vi "GetSpeedProperties.vi"(11 "properties":T2[](array[typedef])) -> (1 "speed reference id":string, 2 "nominal speed":dbl, 3 "speed type":T1)   [LabVIEW 2017, in "VibrationAnalysis.lvlib"]
uses:
  <vilib>/addons/InsightCM/Devices/Shared/VibrationAnalysis/VibrationAnalysis.lvlib
  <vilib>/addons/InsightCM/Utilities/PropertyHelpers/PropertyHelpers.lvlib
  <vilib>/addons/InsightCM/Utilities/Analysis/Shared/controls/SpeedType.ctl
  <vilib>/addons/InsightCM/Utilities/Analysis/Shared/AnalysisHelper.lvlib
  <vilib>/addons/InsightCM/MessageBus/Base/controls/KeyValuePair.ctl
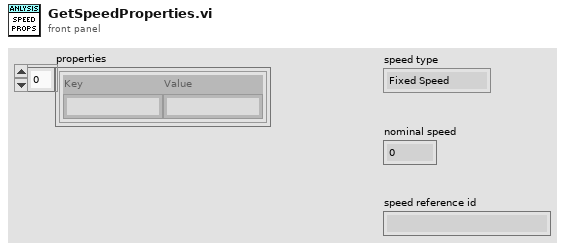
[diagram p1: front panel]
types:
  T1 = typedef "AnalysisHelper.lvlib/SpeedType.ctl" = enum16{"Fixed Speed", "Tachometer"}
  T2 = typedef "KeyValuePair.ctl" = cluster{"Key":string, "Value":string}
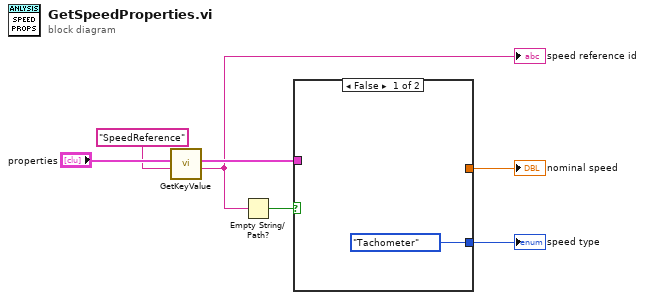
[diagram p0: block diagram]
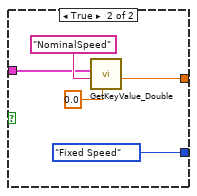
[diagram p2: hidden frame]
diagram:
  n1 = call <vilib>:"GetKeyValue.vi"("key"="SpeedReference", "key value pairs"="properties") -> ("value"=w4:string, "key value pairs out"=w5:T2[])  [unwired: 7 in, 1 out]
  "speed reference id" <- w4
  n2 = Empty String/Path?(string/path=w4) -> (empty?=w3:bool)
  n3 = case shown="False" w3 {
    tunnel: w5 -> [_ w12]
    tunnel: [_ w10] -> w2
    tunnel: [SpeedType."Tachometer" ("Speed Type") SpeedType."Fixed Speed" ("Speed Type")] -> w1
    frame False {
    }
    frame True {
      n4 = call <vilib>:"GetKeyValue_Double.vi"("default"=0.0, "key"="NominalSpeed", "key value pairs"=w12) -> ("value"=w10:dbl)  [unwired: 6 in, 2 out]
    }
  }
  "nominal speed" <- w2
  "speed type" <- w1
